vi "Create build_all.bat.vi"(7 "template folder":path, 8 "error in (no error)":errorcluster, 11 "repository paths":path[](array[path])) -> (0 "error out":errorcluster, 2 "resulting string":string, 3 "build_all.bat path":path)   [LabVIEW 2019, in "Build.lvlib"]
uses:
  Build.lvlib
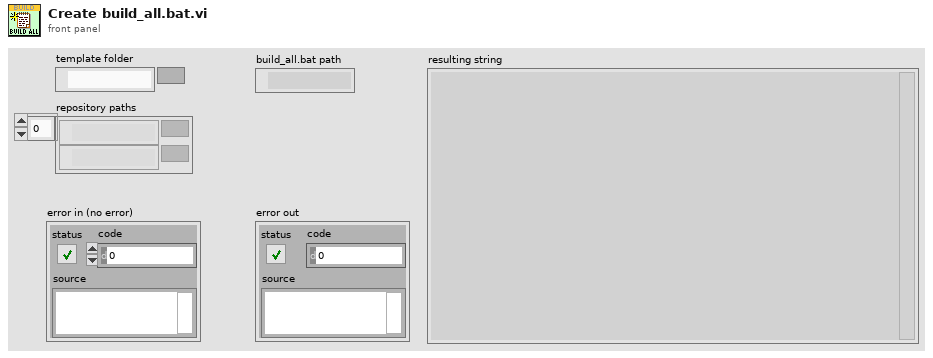
[diagram p1: front panel]
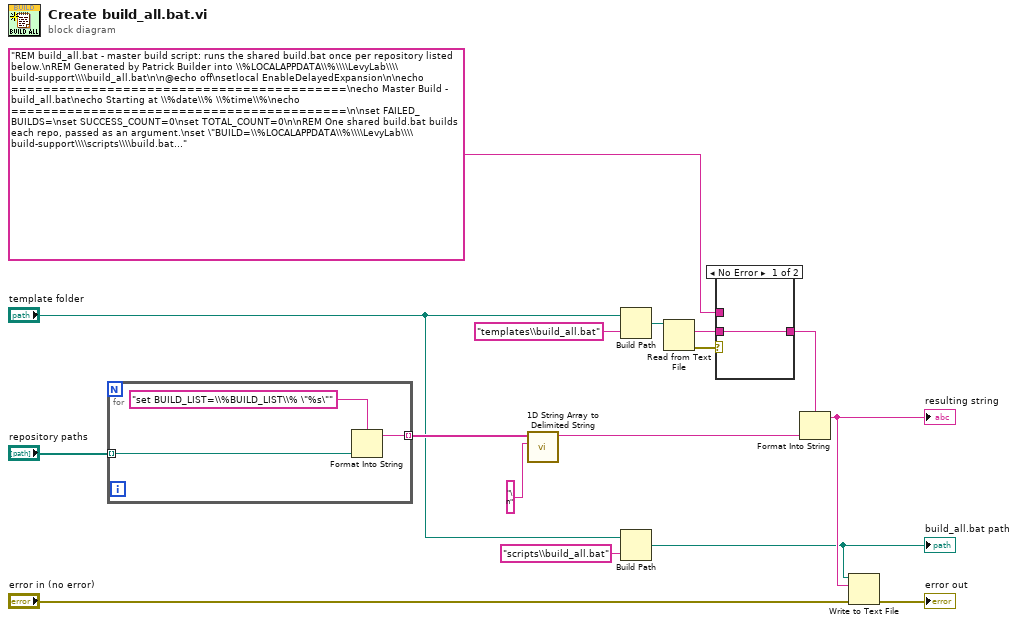
[diagram p0: block diagram]
diagram:
  n1 = for {
    tunnel: [w17] -> w9 mode=indexing
    tunnel: "repository paths" -> [w18] mode=indexing
    n2 = Format Into String(format string="set BUILD_LIST=\\%BUILD_LIST\\% \"%s\"" ("name or relative path"), w18) -> (resulting string=w17:string)  [unwired: 2 in, 1 out]
  }
  n3 = call <vilib>:"1D String Array to Delimited String.vi"("delimiter"="\n", "string array"=w9) -> ("delimited string"=w7:string)  [unwired: 9 in]
  n4 = Build Path(base path="template folder", name or relative path="templates\\build_all.bat") -> (appended path=w16:path)
  n5 = Build Path(base path="template folder", name or relative path="scripts\\build_all.bat") -> (appended path=w13:path)
  "build_all.bat path" <- w13
  n6 = Read from Text File(file (use dialog)=w16) -> (text=w4:string, error out=w6:errorcluster)  [unwired: 3 in, 2 out]
  n7 = case shown="No Error" w6 {
    tunnel: [w20 w21] -> w5
    tunnel: w4 -> [w20 _]
    tunnel: "REM build_all.bat - master build script: runs the shared build.bat once per repository listed below.\nREM Generated by Patrick Builder into \\%LOCALAPPDATA\\%\\\\LevyLab\\\\build-support\\\\build_all.bat\n\n@echo off\nsetlocal EnableDelayedExpansion\n\necho ==========================================\necho Master Build - build_all.bat\necho Starting at \\%date\\% \\%time\\%\necho ==========================================\n\nset FAILED_BUILDS=\nset SUCCESS_COUNT=0\nset TOTAL_COUNT=0\n\nREM One shared build.bat builds each repo, passed as an argument.\nset \"BUILD=\\%LOCALAPPDATA\\%\\\\LevyLab\\\\build-support\\\\scripts\\\\build.bat\"\n\nREM List of repository roots to build.\nset BUILD_LIST=\n%s\n\nREM Execute each build\nfor \\%\\%R in (\\%BUILD_LIST\\%) do (\n    set /a TOTAL_COUNT+=1\n    set \"REPO_NAME=\\%\\%~nxR\"\n\n    echo.\n    echo ==========================================\n    echo [!TOTAL_COUNT!] Building !REPO_NAME!\n    echo ==========================================\n\n    call \"\\%BUILD\\%\" \"\\%\\%~R\"\n\n    if !ERRORLEVEL! neq 0 (\n        echo ERROR: !REPO_NAME! failed\n        set FAILED_BUILDS=!FAILED_BUILDS! !REPO_NAME!\n    ) else (\n        echo SUCCESS: !REPO_NAME!\n        set /a SUCCESS_COUNT+=1\n    )\n)\n\nREM Summary\necho.\necho ==========================================\necho Build Summary\necho ==========================================\necho Total: \\%TOTAL_COUNT\\%\necho Success: \\%SUCCESS_COUNT\\%\n\nif \"\\%FAILED_BUILDS\\%\"==\"\" (\n    echo All builds completed successfully!\n    exit /b 0\n) else (\n    echo Failed builds:\\%FAILED_BUILDS\\%\n    exit /b 1\n)" -> [_ w21]
    frame No Error {
    }
    frame Error {
    }
  }
  n8 = Format Into String(format string=w5, w7) -> (resulting string=w14:string)  [unwired: 2 in, 1 out]
  "resulting string" <- w14
  n9 = Write to Text File(file (use dialog)=w13, text=w14, error in="error in (no error)") -> (error out=→"error out":errorcluster)  [unwired: 1 in, 2 out]
